vi "Backpack.vi"(7 "JPG":refnum<vi>, 10 "queueName":string="PV_script", 11 "Console Reference":refnum<vi>) -> ()   [LabVIEW 2022 SP3]
panel:
  in  "Read file":bool
  in  "Load File":bool
  in  "Load":bool
  out "Spike":string
  out "Dongle":string
  in  "Send to backpack":string
  in  "Send":bool
  in  "Clear":bool
  in  "Ctrl C":bool
  in  "start":bool
  # "Backpack View"
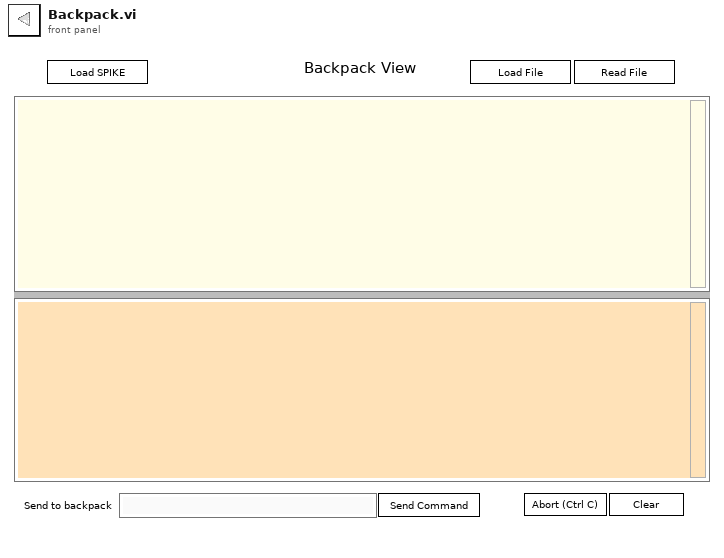
[diagram p1: front panel]
types:
  T1 = enum16{"read", "write pause", "write port", "write path", "write all"}
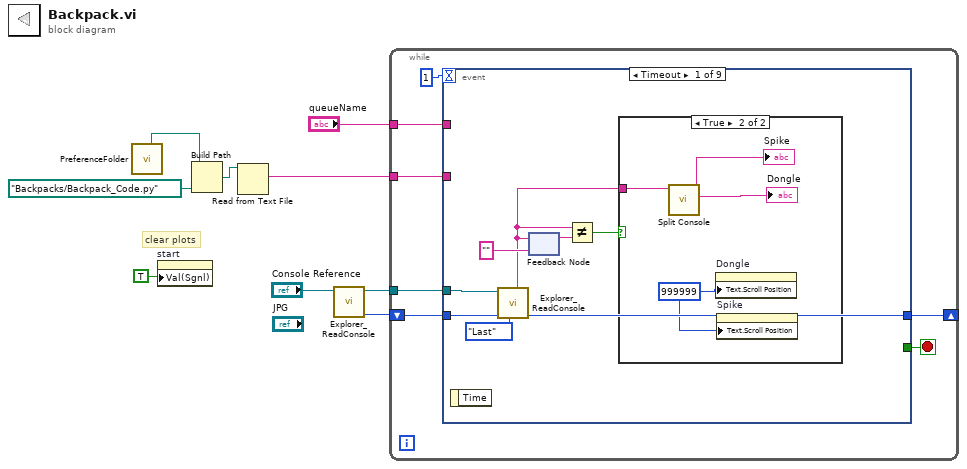
[diagram p0: block diagram]
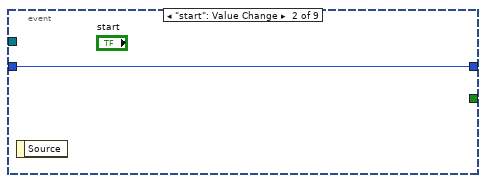
[diagram p3: hidden frame]
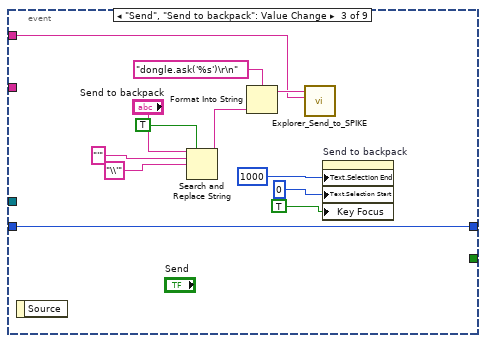
[diagram p4: hidden frame]
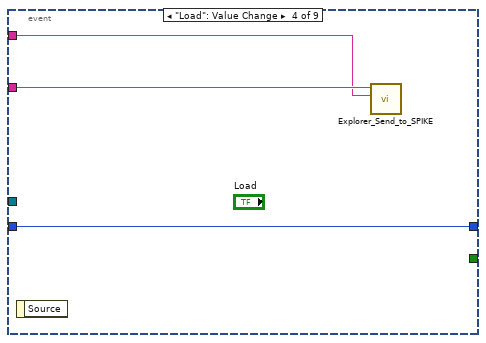
[diagram p5: hidden frame]
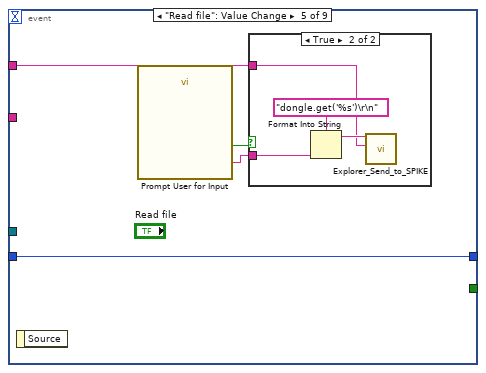
[diagram p6: hidden frame]
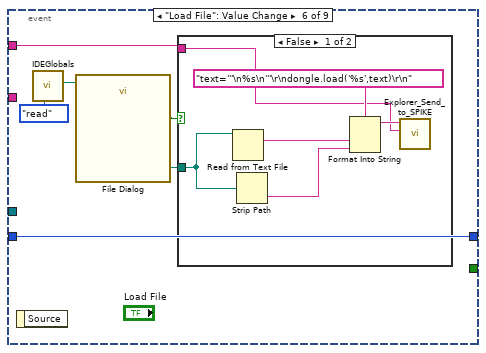
[diagram p8: hidden frame]
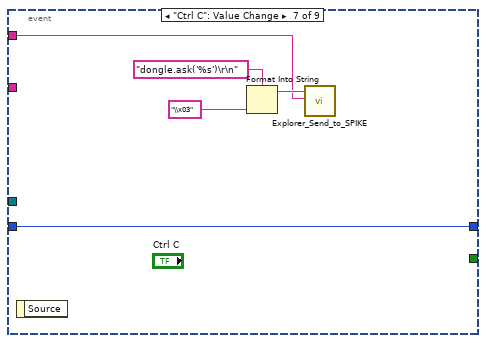
[diagram p10: hidden frame]
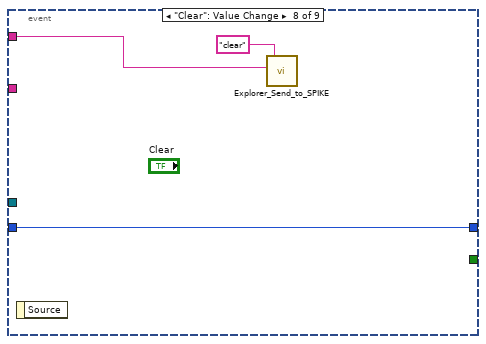
[diagram p11: hidden frame]
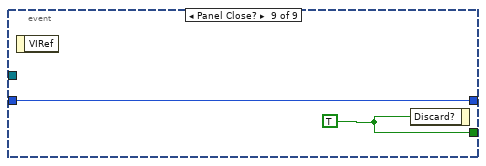
[diagram p12: hidden frame]
diagram:
  # "clear plots"
  n1 = call "PreferenceFolder.vi"() -> ("Examples"=w4:path)  [unwired: 4 in, 7 out]
  n2 = property on="start" class="Bool (strict)"("Val(Sgnl)"=TRUE ("Value (Signaling)")) -> ()  [unwired: 2 in, 2 out]
  n3 = Build Path(base path=w4, name or relative path=path "Backpacks/Backpack_Code.py") -> (appended path=w3:path)
  n4 = Read from Text File(file (use dialog)=w3) -> (text=w2:string)  [unwired: 3 in, 3 out]
  n5 = call "Explorer_ReadConsole.vi"("String in"="Console Reference") -> ("index out"=w8:i32, "String out"=w7:refnum<vi>)  [unwired: 6 in, 3 out]
  n6 = while {
    shift-right: [w14] -> _
    shift-left: w8 -> [w13]
    tunnel: w7 -> [w12]
    tunnel: w2 -> [w11]
    tunnel: "queueName" -> [w10]
    stop <- w15 stop-if-true
    n7 = event shown="[0] Timeout" {
      selector: _ -> [_ _ _ _ _ _ _ _ _]
      dyn-events: _ -> [_ _ _ _ _ _ _ _ _]
      timeout: 1 -> [_ _ _ _ _ _ _ _ _]
      tunnel: [_ _ _ _ _ _ _ _ w74] -> w15
      tunnel: [w23 w29 w41 w44 w48 w58 w69 w72 w73] -> w14
      tunnel: w13 -> [w24 w29 w41 w44 w48 w58 w69 w72 w73]
      tunnel: w12 -> [w22 _ _ _ _ _ _ _ _]
      tunnel: w11 -> [_ _ _ w43 _ _ _ _ _]
      tunnel: w10 -> [_ _ w30 w42 w45 w53 w65 w70 _]
      event Timeout {
        n8 = event-data() -> ()  [unwired: 1 in, 1 out]
        n9 = call "Explorer_ReadConsole.vi"("Reading"=enum16{"Next", "Last"}."Last" ("type"), "index in"=w24, "String in"=w22) -> ("index out"=w23:i32, "Value"=w18:string)  [unwired: 4 in, 3 out]
        n10 = feedback-in #1(w18) -> ()
        n11 = feedback #1("" ("Value")) -> (w19:string)
        n12 = Not Equal?(x=w18, y=w19) -> (x != y?=w17:bool)
        n13 = case shown="True" w17 {
          tunnel: w18 -> [_ w28]
          frame False {
          }
          frame True {
            w25 = u32 999999 ("Text.Scroll Position")
            n14 = call "Split Console.vi"("Console"=w28) -> ("Dongle"=→"Dongle":string, "Spike"=→"Spike":string)  [unwired: 9 in]
            n15 = property on="Dongle" class="Str"("Text.Scroll Position"=w25) -> ()  [unwired: 2 in, 2 out]
            n16 = property on="Spike" class="Str"("Text.Scroll Position"=w25) -> ()  [unwired: 2 in, 2 out]
          }
        }
      }
      event "start": Value Change {
        n17 = event-data() -> ()  [unwired: 1 in, 1 out]
      }
      event "Send", "Send to backpack": Value Change {
        n18 = event-data() -> ()  [unwired: 1 in, 1 out]
        n19 = Search and Replace String(replace all?=TRUE ("replace all? (F)"), input string="Send to backpack", search string="'" ("string"), replace string="\\'" ("string")) -> (result string=w34:string)  [unwired: 4 in, 3 out]
        n20 = Format Into String(format string="dongle.ask('%s')\r\n" ("string"), w34) -> (resulting string=w39:string)  [unwired: 2 in, 1 out]
        n21 = call "Explorer_Send_to_SPIKE.vi"("queueName"=w30, "python"=w39) -> ()  [unwired: 9 in, 1 out]
        n22 = property on="Send to backpack" class="Str"("Text.Selection End"=u32 1000 ("Selection Start"), "Text.Selection Start"=u32 0 ("Selection End"), "Key Focus"=TRUE) -> ()  [unwired: 2 in, 2 out]
      }
      event "Load": Value Change {
        n23 = event-data() -> ()  [unwired: 1 in, 1 out]
        n24 = call "Explorer_Send_to_SPIKE.vi"("queueName"=w42, "python"=w43) -> ()  [unwired: 9 in, 1 out]
      }
      event "Read file": Value Change {
        n25 = event-data() -> ()  [unwired: 1 in, 1 out]
        n26 = call "Prompt User for Input"() -> ("filename"=w46:string, "OK"=w47:bool)  [unwired: 17 in, 1 out]
        n27 = case shown="True" w47 {
          tunnel: w46 -> [_ w52]
          tunnel: w45 -> [_ w49]
          frame False {
          }
          frame True {
            n28 = Format Into String(format string="dongle.get('%s')\r\n", w52) -> (resulting string=w50:string)  [unwired: 2 in, 1 out]
            n29 = call "Explorer_Send_to_SPIKE.vi"("queueName"=w49, "python"=w50) -> ()  [unwired: 9 in, 1 out]
          }
        }
      }
      event "Load File": Value Change {
        n30 = event-data() -> ()  [unwired: 1 in, 1 out]
        n31 = call "IDEGlobals.vi"("task"=T1."read") -> ("Last Path out"=w55:path)  [unwired: 8 in, 2 out]
        n32 = call "File Dialog"("start path"=w55) -> ("selected path"=w56:path, "cancelled"=w57:bool)  [unwired: 11 in, 2 out]
        n33 = case shown="False" w57 {
          tunnel: w56 -> [w62 _]
          tunnel: w53 -> [w59 _]
          frame False {
            n34 = Read from Text File(file (use dialog)=w62) -> (text=w61:string)  [unwired: 3 in, 3 out]
            n35 = Strip Path(path=w62) -> (name=w60:string)  [unwired: 1 out]
            n36 = Format Into String(format string="text='''\n%s\n'''\r\ndongle.load('%s',text)\r\n" ("string"), w61, w60) -> (resulting string=w63:string)  [unwired: 2 in, 1 out]
            n37 = call "Explorer_Send_to_SPIKE.vi"("queueName"=w59, "python"=w63) -> ()  [unwired: 9 in, 1 out]
          }
          frame True {
          }
        }
      }
      event "Ctrl C": Value Change {
        n38 = event-data() -> ()  [unwired: 1 in, 1 out]
        n39 = Format Into String(format string="dongle.ask('%s')\r\n" ("string"), "\\x03" ("Send to backpack 2")) -> (resulting string=w67:string)  [unwired: 2 in, 1 out]
        n40 = call "Explorer_Send_to_SPIKE.vi"("queueName"=w65, "python"=w67) -> ()  [unwired: 9 in, 1 out]
      }
      event "Clear": Value Change {
        n41 = event-data() -> ()  [unwired: 1 in, 1 out]
        n42 = call "Explorer_Send_to_SPIKE.vi"("queueName"=w70, "python"="clear" ("string")) -> ()  [unwired: 9 in, 1 out]
      }
      event Panel Close? {
        w74 = TRUE ("Discard?")
        n43 = event-data() -> ()  [unwired: 1 in, 1 out]
        n44 = event-data("Discard?"=w74) -> ()  [unwired: 1 in, 1 out]
      }
    }
  }
